vi "ConfigureSource.vi"(7 "SMU":T1, 8 "Error In":errorcluster, 10 "Source Configuration":T2, 11 "Keithley 2602 In":refnum<visa-resource-name>) -> (0 "Error Out":errorcluster, 3 "Keithley 2602 Out":refnum<visa-resource-name>)   [LabVIEW 2013]
uses:
  SourceConfiguration.ctl
  SourceFunction.ctl
  driver/Public/Controls/SMU.ctl
  driver/Public/Controls/DisplayFunction.ctl
  driver/Public/Controls/SourceFunction.ctl
  driver/Keithley-2602.lvlib
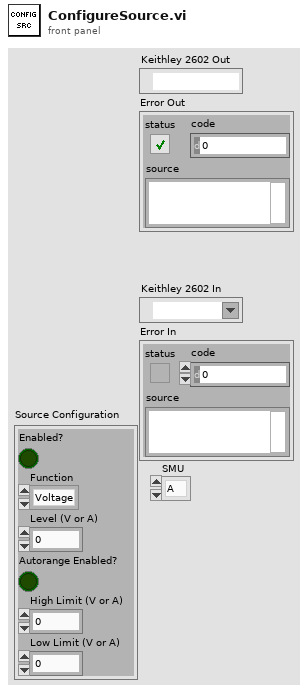
[diagram p1: front panel]
types:
  T1 = typedef "Keithley-2602.lvlib/SMU.ctl" = enum16{"A", "B"}
  T2 = typedef "SourceConfiguration.ctl" = cluster{"Enabled?":bool, "Function":T3, "Level (V or A)":dbl, "Autorange Enabled?":bool, "High Limit (V or A)":dbl, "Low Limit (V or A)":dbl}
  T3 = typedef "SourceFunction.ctl" = enum16{"Voltage", "Current"}
  T4 = typedef "Keithley-2602.lvlib/SourceFunction.ctl" = enum16{"Voltage", "Current"}
  T5 = typedef "Keithley-2602.lvlib/DisplayFunction.ctl" = enum16{"Current", "Voltage", "Resistance", "Power"}
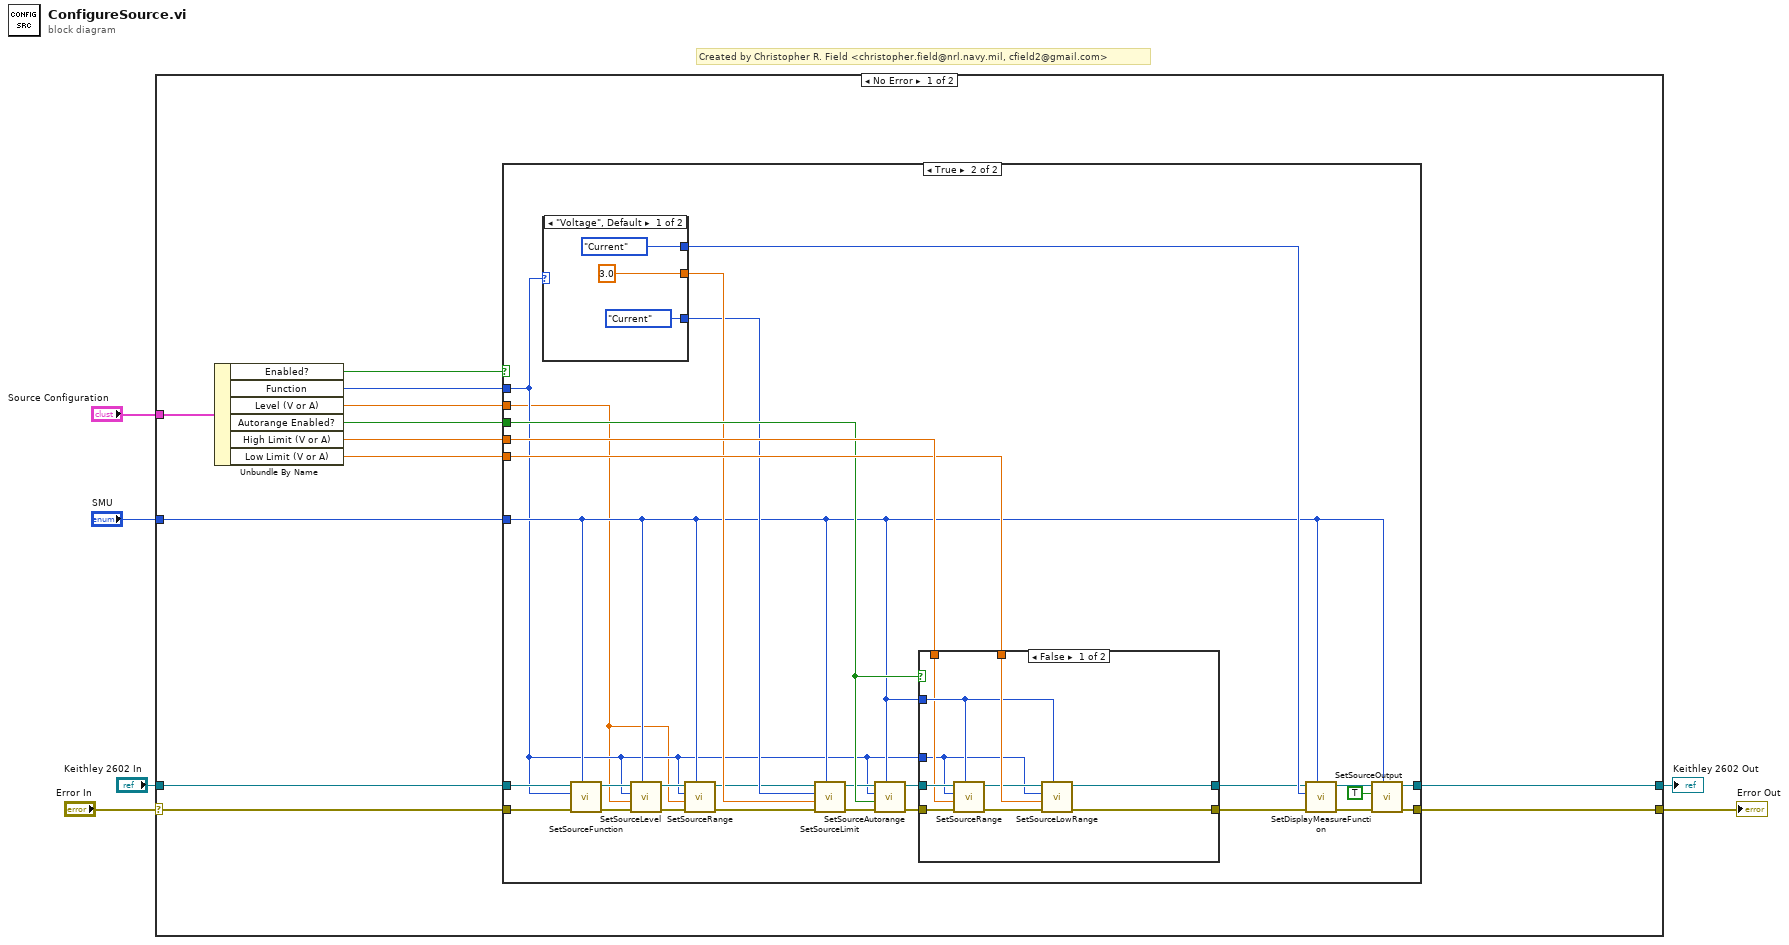
[diagram p0: block diagram]
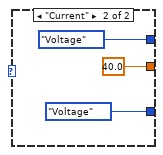
[diagram p4: hidden frame]
diagram:
  # "Created by Christopher R. Field <christopher.field@nrl.navy.mil, cfield2@gmail.com>"
  n1 = case shown="No Error" "Error In" {
    selector: "Error In" -> [w17 w67]
    tunnel: "Source Configuration" -> [w16 _]
    tunnel: "Keithley 2602 In" -> [w18 w68]
    tunnel: "SMU" -> [w12 _]
    tunnel: [w8 w68] -> w2
    tunnel: [w7 w67] -> w1
    frame No Error {
      n2 = Unbundle By Name(w16) -> ("Enabled?"=w15:bool, "Function"=w14:T3, "Level (V or A)"=w13:dbl, "Autorange Enabled?"=w11:bool, "High Limit (V or A)"=w10:dbl, "Low Limit (V or A)"=w9:dbl)
      n3 = case shown="True" w15 {
        tunnel: w18 -> [w20 w42]
        tunnel: w17 -> [w19 w41]
        tunnel: w14 -> [_ w22]
        tunnel: w13 -> [_ w21]
        tunnel: w12 -> [_ w26]
        tunnel: w11 -> [_ w34]
        tunnel: w10 -> [_ w39]
        tunnel: w9 -> [_ w37]
        tunnel: [w20 w33] -> w8
        tunnel: [w19 w32] -> w7
        frame False {
        }
        frame True {
          n4 = case shown="\"Voltage\", Default" w22 {
            tunnel: [DisplayFunction."Current" ("Display Function") DisplayFunction."Voltage" ("Display Function")] -> w43
            tunnel: [3.0 40.0] -> w29
            tunnel: [SourceFunction."Current" ("Source Function") SourceFunction."Voltage" ("Source Function")] -> w28
            frame "Voltage", Default {
            }
            frame "Current" {
            }
          }
          n5 = call "SetSourceFunction.vi"("SMU"=w26, "Error In"=w41, "Source Function"=w22, "Keithley 2602 In"=w42) -> ("Error Out"=w47:errorcluster, "Keithley 2602 Out"=w48:refnum<visa-resource-name>)  [unwired: 6 in]
          n6 = call "SetSourceLevel.vi"("SMU"=w26, "Error In"=w47, "Level (V or A)"=w21, "Source Function"=w22, "Keithley 2602 In"=w48) -> ("Error Out"=w23:errorcluster, "Keithley 2602 Out"=w27:refnum<visa-resource-name>)  [unwired: 5 in]
          n7 = call "SetSourceRange.vi"("SMU"=w26, "Error In"=w23, "Range (V or A)"=w21, "Source Function"=w22, "Keithley 2602 In"=w27) -> ("Error Out"=w24:errorcluster, "Keithley 2602 Out"=w25:refnum<visa-resource-name>)  [unwired: 5 in]
          n8 = call "SetSourceLimit.vi"("SMU"=w26, "Error In"=w24, "Limit (V or A)"=w29, "Source Function"=w28, "Keithley 2602 In"=w25) -> ("Error Out"=w30:errorcluster, "Keithley 2602 Out"=w31:refnum<visa-resource-name>)  [unwired: 5 in]
          n9 = call "SetSourceAutorange.vi"("SMU"=w26, "Error In"=w30, "Enable?"=w34, "Source Function"=w22, "Keithley 2602 In"=w31) -> ("Error Out"=w38:errorcluster, "Keithley 2602 Out"=w40:refnum<visa-resource-name>)  [unwired: 5 in]
          n10 = case shown="False" w34 {
            tunnel: w40 -> [w55 w60]
            tunnel: w39 -> [w50 _]
            tunnel: w38 -> [w54 w59]
            tunnel: w37 -> [w58 _]
            tunnel: w22 -> [w49 _]
            tunnel: w26 -> [w51 _]
            tunnel: [w57 w60] -> w36
            tunnel: [w56 w59] -> w35
            frame False {
              n11 = call "SetSourceRange.vi"("SMU"=w51, "Error In"=w54, "Range (V or A)"=w50, "Source Function"=w49, "Keithley 2602 In"=w55) -> ("Error Out"=w52:errorcluster, "Keithley 2602 Out"=w53:refnum<visa-resource-name>)  [unwired: 5 in]
              n12 = call "SetSourceLowRange.vi"("SMU"=w51, "Error In"=w52, "Low Range (V or A)"=w58, "Source Function"=w49, "Keithley 2602 In"=w53) -> ("Error Out"=w56:errorcluster, "Keithley 2602 Out"=w57:refnum<visa-resource-name>)  [unwired: 5 in]
            }
            frame True {
            }
          }
          n13 = call "SetDisplayMeasureFunction.vi"("SMU"=w26, "Error In"=w35, "Display Function"=w43, "Keithley 2602 In"=w36) -> ("Error Out"=w44:errorcluster, "Keithley 2602 Out"=w45:refnum<visa-resource-name>)  [unwired: 6 in]
          n14 = call "SetSourceOutput.vi"("SMU"=w26, "Error In"=w44, "Enable?"=TRUE, "Keithley 2602 In"=w45) -> ("Error Out"=w32:errorcluster, "Keithley 2602 Out"=w33:refnum<visa-resource-name>)  [unwired: 6 in]
        }
      }
    }
    frame Error {
    }
  }
  "Keithley 2602 Out" <- w2
  "Error Out" <- w1
